vi "Query Questionable Condition Register.vi"(8 "error in":errorcluster, 10 "Status in":T1, 11 "6032A in":refnum<class "6032A.lvclass">) -> (0 "error out":errorcluster, 2 "Status out":T1, 3 "6032A out":refnum<class "6032A.lvclass">)   [LabVIEW 2019, in "6032A.lvlib" / "6032A.lvclass"]
uses:
  Library/6032A.lvclass
  builds/Instruments/PowerSupply.lvlibp/Custom Controls/Status_Flags.ctl
  Library/6032A.lvclass/6032A.ctl
  builds/Instruments/PowerSupply.lvlibp/Library/PowerSupply.lvclass
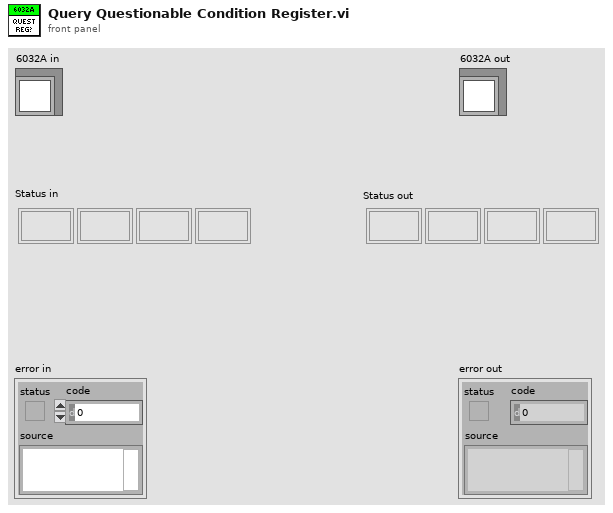
[diagram p1: front panel]
types:
  T1 = typedef "PowerSupply.lvlibp/PowerSupply.lvclass/Status_Flags.ctl" = cluster{"Interlock":bool, "OVP":bool, "OCP":bool, "Output":bool}
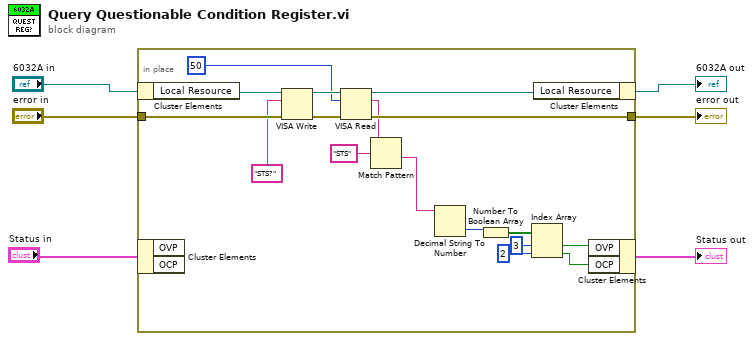
[diagram p0: block diagram]
diagram:
  n1 = in-place {
    in-place-border: [w19] -> w4
    in-place-border: "error in" -> [w18]
    n2 = in-place-cluster #1("6032A in") -> ("Local Resource"=w23:refnum<visa-resource-name>)
    n3 = in-place-cluster #2("Status in") -> ()  [unwired: 2 out]
    n4 = VISA Write(VISA resource name=w23, write buffer="STS?", error in (no error)=w18) -> (VISA resource name out=w22:refnum<visa-resource-name>, error out=w20:errorcluster)  [unwired: 1 out]
    n5 = VISA Read(VISA resource name=w22, byte count=u32 50, error in (no error)=w20) -> (VISA resource name out=w21:refnum<visa-resource-name>, read buffer=w15:string, error out=w19:errorcluster)  [unwired: 1 out]
    n6 = Match Pattern(string=w15, regular expression="STS") -> (after substring=w8:string)  [unwired: 1 in, 3 out]
    n7 = Decimal String To Number(string=w8) -> (number=w14:i32)  [unwired: 2 in, 1 out]
    n8 = Number To Boolean Array(number=w14) -> (Boolean array=w13:bool[])
    n9 = Index Array(array=w13, index #1=3 ("index"), index #2=2 ("index")) -> (element #1=w10:bool, element #2=w9:bool)
    n10 = in-place-cluster #1("Local Resource"=w21) -> (→"6032A out":refnum<class "6032A.lvclass">)
    n11 = in-place-cluster #2("OVP"=w10, "OCP"=w9) -> (→"Status out":T1)
  }
  "error out" <- w4
